vi "Brute Force Dark Current Primary Logic Body.vi"(0 "Barcodes in":string[](array[string]), 1 "stop":bool, 2 "Data Pin in":refnum<k21>, 3 "Sync Pin in":refnum<k21>, 4 "Write Pin in":refnum<k21>, 5 "Clear Pin in":refnum<k21>, 6 "Number of Tubes":i32, 7 "Channel #":i32, 8 "Trip Count":dbl) -> (10 "Actual Voltage Level (V)":dbl format="%#_13g", 11 "Individual Tube Current (Nano Amps)":dbl[](array[numeric]), 12 "Actual Current Limit (nA)":dbl format="%#_13g", 13 "Mesurnment Iteration":i32, 14 "Power Supply Trip":bool, 15 "Data Pin out":refnum<k21>, 16 "Sync Pin out":refnum<k21>, 17 "Write Pin out":refnum<k21>, 18 "Clear Pin out":refnum<k21>, 19 "Failed Tubes":string[](array[string]))   [LabVIEW 2020]
uses:
  <instrlib>/CAEN PSM/CAEN PSM.lvlib
panel:
  out "BoardHandle out":T1
  out "error out":errorcluster
  in  "VISA Refnum in":refnum<visa-resource-name>
  # "Pin in"
  # "Pin out"
  # "No pin"
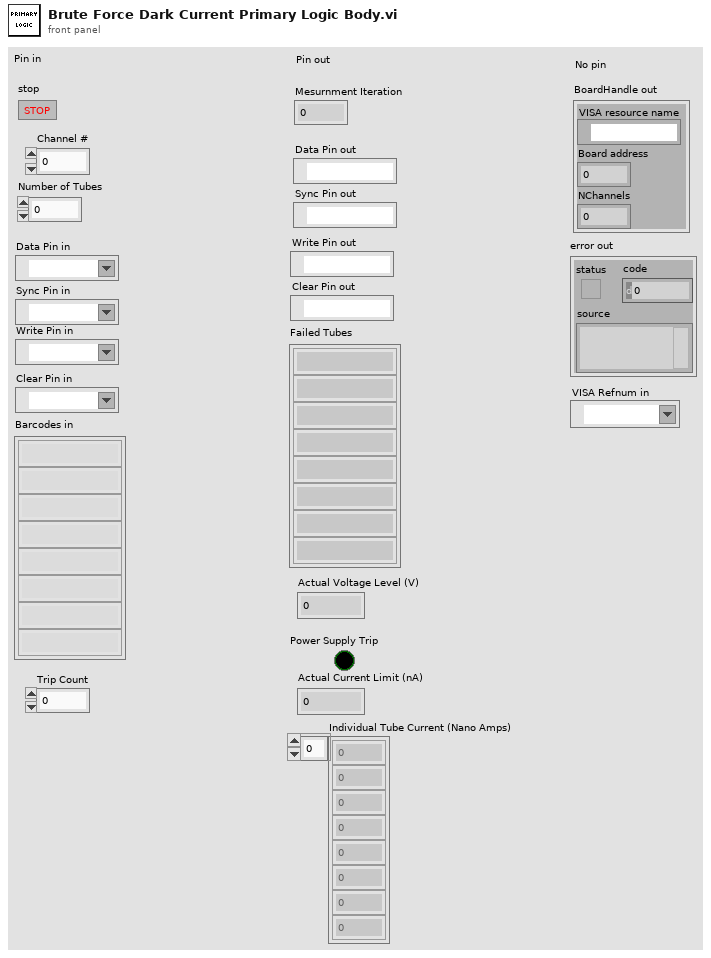
[diagram p1: front panel]
types:
  T1 = cluster{"VISA resource name":refnum<visa-resource-name>, "Board address":u8, "NChannels":u8}
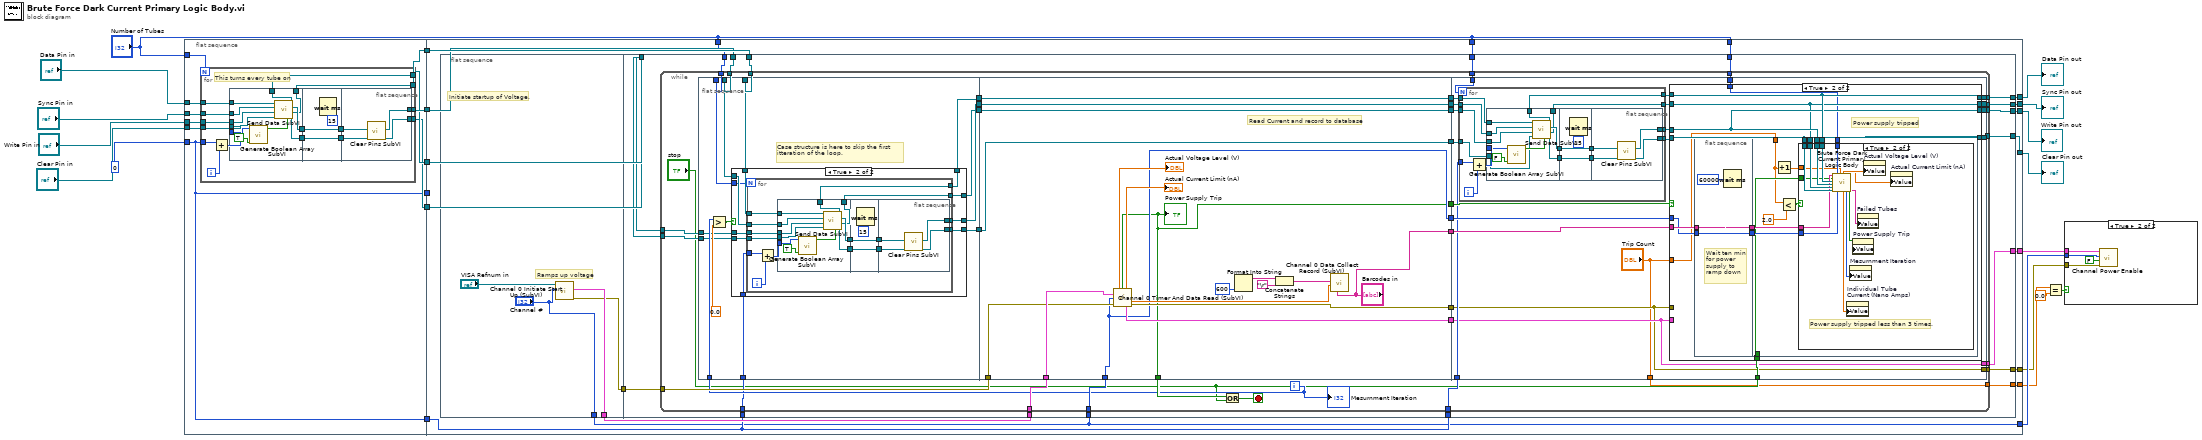
[diagram p0: block diagram]
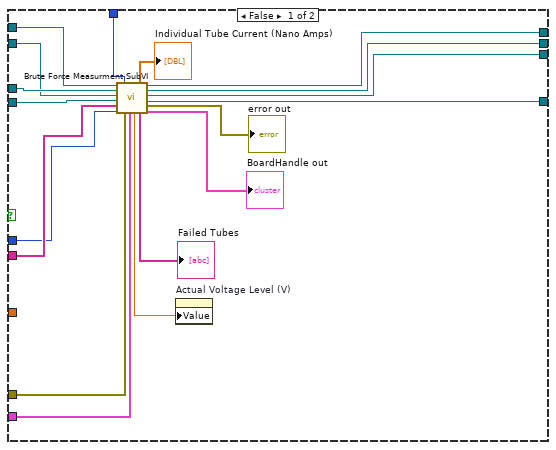
[diagram p4: hidden frame]
diagram:
  n1 = flat-sequence {
    tunnel: 0 ("First Tube #") -> [w23]
    tunnel: "Number of Tubes" -> [w29]
    tunnel: "Data Pin in" -> [w32]
    tunnel: "Sync Pin in" -> [w31]
    tunnel: "Write Pin in" -> [w30]
    tunnel: [w23] -> w22
    tunnel: "Clear Pin in" -> [w28]
    tunnel: [w27] -> w16
    tunnel: [w26] -> w15
    tunnel: [w25] -> w14
    tunnel: [w24] -> w13
    tunnel: [w23] -> w11
    tunnel: w22 -> [w70]
    tunnel: "Number of Tubes" -> [w83]
    tunnel: w16 -> [w80]
    tunnel: w15 -> [w79]
    tunnel: w14 -> [w78]
    tunnel: w13 -> [w77]
    tunnel: "Number of Tubes" -> [w82]
    tunnel: "Number of Tubes" -> [w76]
    tunnel: w11 -> [_]
    tunnel: [w74] -> w10
    tunnel: [w73] -> w9
    tunnel: [w72] -> w8
    tunnel: [w71] -> w7
    tunnel: [w69] -> w6
    tunnel: [w68] -> w5
    tunnel: [w67] -> w4
    tunnel: [w66] -> w2
    frame #0 {
      n2 = for {
        N: w29 -> [_]
        tunnel: w32 -> [w47]
        tunnel: w31 -> [w46]
        tunnel: w30 -> [w45]
        tunnel: [w44] -> w26
        tunnel: [w43] -> w24
        tunnel: [w42] -> w25
        tunnel: [w41] -> w27
        tunnel: w23 -> [w38]
        tunnel: w28 -> [w37]
        i -> [w39]
        # "This turns every tube on"
        n3 = Add(x=w38, y=w39) -> (x+y=w40:i32)
        n4 = flat-sequence {
          tunnel: w40 -> [w56]
          tunnel: w47 -> [w55]
          tunnel: w46 -> [w54]
          tunnel: w45 -> [w53]
          tunnel: [w52] -> w36
          tunnel: [w51] -> w34
          tunnel: [w50] -> w42
          tunnel: [w49] -> w41
          tunnel: w37 -> [w48]
          tunnel: w36 -> [w61]
          tunnel: [w61] -> w35
          tunnel: w34 -> [w60]
          tunnel: [w60] -> w33
          tunnel: w35 -> [w65]
          tunnel: w33 -> [w64]
          tunnel: [w63] -> w44
          tunnel: [w62] -> w43
          frame #0 {
            n5 = call "Generate Boolean Array SubVI.vi"("Activate: 1\nDeactivate: 0"=TRUE, "Tube"=w56) -> ("Boolean array"=w57:bool[])  [unwired: 9 in]
            n6 = call "Send Data SubVI.vi"("Data Pin Task In"=w55, "Sync Pin Task In"=w54, "Write Pin Task In"=w53, "Clear Pin Task In"=w48, "Data"=w57) -> ("Data Pin Task Out"=w49:refnum<k21>, "Sync Pin Task Out"=w52:refnum<k21>, "Write Pin Task Out"=w50:refnum<k21>, "Clear Pin Task Out"=w51:refnum<k21>)  [unwired: 1 in]
          }
          frame #1 {
            n7 = Wait (ms)(milliseconds to wait=u32 15) -> ()  [unwired: 1 out]
          }
          frame #2 {
            n8 = call "Clear Pins SubVI.vi"("Clear Pin Task In"=w64, "Sync Pin Task In"=w65) -> ("Clear Pin Task Out"=w62:refnum<k21>, "Sync Pin Task Out"=w63:refnum<k21>)  [unwired: 8 in]
          }
        }
      }
    }
    frame #1 {
      n9 = flat-sequence {
        tunnel: ["Channel #"] -> w69
        tunnel: [w86] -> w81
        tunnel: [w84] -> w75
        tunnel: w83 -> [w106]
        tunnel: w70 -> [w105]
        tunnel: w82 -> [w104]
        tunnel: w69 -> [w103]
        tunnel: w81 -> [w102]
        tunnel: w80 -> [w101]
        tunnel: w79 -> [w100]
        tunnel: w78 -> [w99]
        tunnel: w77 -> [w98]
        tunnel: w76 -> [w97]
        tunnel: w75 -> [w96]
        tunnel: [w95] -> w71
        tunnel: [w94] -> w72
        tunnel: [w93] -> w73
        tunnel: [w92] -> w74
        tunnel: w70 -> [w91]
        tunnel: [w90] -> w68
        tunnel: [w89] -> w67
        tunnel: [w88] -> w66
        frame #0 {
          # "Ramps up voltage"
          # "Initiate startup of Voltage."
          n10 = call "Channel 0 Initiate Start Up (SubVI).vi"("Channel # in"="Channel #", "VISA Refnum in"="VISA Refnum in") -> ("error out"=w84:errorcluster, "BoardHandle out"=w86:T1)  [unwired: 8 in]
        }
        frame #1 {
          n11 = while {
            tunnel: w106 -> [w142]
            tunnel: w105 -> [w141]
            tunnel: w104 -> [w140]
            tunnel: w103 -> [w139]
            tunnel: w102 -> [w138]
            tunnel: w101 -> [w137]
            tunnel: w100 -> [w136]
            tunnel: w99 -> [w135]
            tunnel: w98 -> [w134]
            tunnel: w97 -> [w125]
            tunnel: w96 -> [w120]
            tunnel: [w119] -> w95
            tunnel: [w118] -> w94
            tunnel: [w117] -> w93
            tunnel: [w116] -> w92
            tunnel: w91 -> [w112]
            tunnel: [w109] -> w90
            tunnel: [w108] -> w89
            tunnel: [w107] -> w88
            i -> [w113]
            stop <- w114 stop-if-true
            n12 = flat-sequence {
              tunnel: w113 -> [w153]
              tunnel: w137 -> [w152]
              tunnel: w136 -> [w151]
              tunnel: w135 -> [w150]
              tunnel: w134 -> [w149]
              tunnel: [w148] -> w132
              tunnel: [w147] -> w130
              tunnel: [w146] -> w128
              tunnel: [w145] -> w126
              tunnel: w125 -> [w144]
              tunnel: w112 -> [w143]
              tunnel: w139 -> [w204]
              tunnel: w138 -> [w207]
              tunnel: [w215] -> w133
              tunnel: w132 -> [w215]
              tunnel: [w214] -> w131
              tunnel: w130 -> [w214]
              tunnel: [w213] -> w129
              tunnel: w128 -> [w213]
              tunnel: [w212] -> w127
              tunnel: w126 -> [w212]
              tunnel: [w211] -> w124
              tunnel: [w204] -> w123
              tunnel: [w209] -> w122
              tunnel: ["Barcodes in"] -> w121
              tunnel: w120 -> [w206]
              tunnel: [w203] -> w115
              tunnel: [w203] -> w111
              tunnel: w142 -> [w240]
              tunnel: [w239] -> w119
              tunnel: [w238] -> w118
              tunnel: [w237] -> w117
              tunnel: [w236] -> w116
              tunnel: w121 -> [w242]
              tunnel: w122 -> [w223]
              tunnel: w123 -> [w241]
              tunnel: w124 -> [w222]
              tunnel: w127 -> [w229]
              tunnel: w129 -> [w230]
              tunnel: w131 -> [w231]
              tunnel: w133 -> [w232]
              tunnel: w140 -> [w234]
              tunnel: w141 -> [w233]
              tunnel: w111 -> [w235]
              tunnel: "stop" -> [w224]
              tunnel: [w223] -> w109
              tunnel: [w222] -> w108
              tunnel: ["Trip Count"] -> w107
              frame #0 {
                # "Case structure is here to skip the first itteration of the loop."
                n13 = Greater?(x=w153, y=0.0) -> (0:w155:bool)
                n14 = case shown="True" w155 {
                  tunnel: w152 -> [w159 w169]
                  tunnel: w151 -> [w158 w168]
                  tunnel: w150 -> [w157 w167]
                  tunnel: w149 -> [w156 w166]
                  tunnel: [w159 w165] -> w148
                  tunnel: [w158 w164] -> w147
                  tunnel: [w157 w163] -> w146
                  tunnel: [w156 w162] -> w145
                  tunnel: w144 -> [_ w161]
                  tunnel: w143 -> [_ w160]
                  frame False {
                  }
                  frame True {
                    n15 = for {
                      N: w161 -> [_]
                      tunnel: w169 -> [w184]
                      tunnel: w168 -> [w183]
                      tunnel: w167 -> [w182]
                      tunnel: [w181] -> w164
                      tunnel: [w180] -> w162
                      tunnel: [w179] -> w163
                      tunnel: [w178] -> w165
                      tunnel: w160 -> [w175]
                      tunnel: w166 -> [w174]
                      i -> [w176]
                      n16 = Add(x=w175, y=w176) -> (x+y=w177:i32)
                      n17 = flat-sequence {
                        tunnel: w177 -> [w193]
                        tunnel: w184 -> [w192]
                        tunnel: w183 -> [w191]
                        tunnel: w182 -> [w190]
                        tunnel: [w189] -> w173
                        tunnel: [w188] -> w171
                        tunnel: [w187] -> w179
                        tunnel: [w186] -> w178
                        tunnel: w174 -> [w185]
                        tunnel: w173 -> [w198]
                        tunnel: [w198] -> w172
                        tunnel: w171 -> [w197]
                        tunnel: [w197] -> w170
                        tunnel: w172 -> [w202]
                        tunnel: w170 -> [w201]
                        tunnel: [w200] -> w181
                        tunnel: [w199] -> w180
                        frame #0 {
                          n18 = call "Generate Boolean Array SubVI.vi"("Activate: 1\nDeactivate: 0"=TRUE, "Tube"=w193) -> ("Boolean array"=w194:bool[])  [unwired: 9 in]
                          n19 = call "Send Data SubVI.vi"("Data Pin Task In"=w192, "Sync Pin Task In"=w191, "Write Pin Task In"=w190, "Clear Pin Task In"=w185, "Data"=w194) -> ("Data Pin Task Out"=w186:refnum<k21>, "Sync Pin Task Out"=w189:refnum<k21>, "Write Pin Task Out"=w187:refnum<k21>, "Clear Pin Task Out"=w188:refnum<k21>)  [unwired: 1 in]
                        }
                        frame #1 {
                          n20 = Wait (ms)(milliseconds to wait=u32 15) -> ()  [unwired: 1 out]
                        }
                        frame #2 {
                          n21 = call "Clear Pins SubVI.vi"("Clear Pin Task In"=w201, "Sync Pin Task In"=w202) -> ("Clear Pin Task Out"=w199:refnum<k21>, "Sync Pin Task Out"=w200:refnum<k21>)  [unwired: 8 in]
                        }
                      }
                    }
                  }
                }
              }
              frame #1 {
                # "Read Current and record to database"
                n22 = call "Channel 0 Timer And Data Read (SubVI).vi"("BoardHandle in"=w207, "Channel # in"=w204, "error in (no error)"=w206) -> ("Actual Voltage Level (V)"=→"Actual Voltage Level (V)":dbl, "Power Supply Trip"=w203:bool, "Actual Current Limit (nA)"=→"Actual Current Limit (nA)":dbl, "Array"=w210:dbl[], "BoardHandle out 2"=w209:T1, "error out"=w211:errorcluster)  [unwired: 7 in]
                "Power Supply Trip" <- w203
                n23 = Format Into String(600 ("input 1")) -> (resulting string=w219:string)  [unwired: 3 in, 1 out]
                n24 = Concatenate Strings(w219, "\r") -> (w220:string)
                n25 = call "Channel 0 Data Collect Record (SubVI).vi"("Barcodes"="Barcodes in", "Array"=w210, "String"=w220) -> ()  [unwired: 9 in]
              }
              frame #2 {
                n26 = for {
                  N: w234 -> [_]
                  tunnel: w232 -> [w257]
                  tunnel: w231 -> [w256]
                  tunnel: w230 -> [w255]
                  tunnel: [w254] -> w226
                  tunnel: [w253] -> w228
                  tunnel: [w252] -> w225
                  tunnel: w233 -> [w248]
                  tunnel: w229 -> [w247]
                  tunnel: [w251] -> w227
                  i -> [w249]
                  n27 = Add(x=w248, y=w249) -> (x+y=w250:i32)
                  n28 = flat-sequence {
                    tunnel: w250 -> [w266]
                    tunnel: w257 -> [w265]
                    tunnel: w256 -> [w264]
                    tunnel: w255 -> [w263]
                    tunnel: [w262] -> w246
                    tunnel: [w261] -> w244
                    tunnel: [w260] -> w252
                    tunnel: [w259] -> w251
                    tunnel: w247 -> [w258]
                    tunnel: w246 -> [w271]
                    tunnel: [w271] -> w245
                    tunnel: w244 -> [w270]
                    tunnel: [w270] -> w243
                    tunnel: w245 -> [w275]
                    tunnel: w243 -> [w274]
                    tunnel: [w273] -> w254
                    tunnel: [w272] -> w253
                    frame #0 {
                      n29 = call "Generate Boolean Array SubVI.vi"("Activate: 1\nDeactivate: 0"=FALSE, "Tube"=w266) -> ("Boolean array"=w267:bool[])  [unwired: 9 in]
                      n30 = call "Send Data SubVI.vi"("Data Pin Task In"=w265, "Sync Pin Task In"=w264, "Write Pin Task In"=w263, "Clear Pin Task In"=w258, "Data"=w267) -> ("Data Pin Task Out"=w259:refnum<k21>, "Sync Pin Task Out"=w262:refnum<k21>, "Write Pin Task Out"=w260:refnum<k21>, "Clear Pin Task Out"=w261:refnum<k21>)  [unwired: 1 in]
                    }
                    frame #1 {
                      n31 = Wait (ms)(milliseconds to wait=u32 15) -> ()  [unwired: 1 out]
                    }
                    frame #2 {
                      n32 = call "Clear Pins SubVI.vi"("Clear Pin Task In"=w274, "Sync Pin Task In"=w275) -> ("Clear Pin Task Out"=w272:refnum<k21>, "Sync Pin Task Out"=w273:refnum<k21>)  [unwired: 8 in]
                    }
                  }
                }
                n33 = case shown="True" w235 {
                  tunnel: w242 -> [w293 w299]
                  tunnel: w241 -> [w292 w298]
                  tunnel: w222 -> [w291 _]
                  tunnel: w240 -> [w290 w300]
                  tunnel: w223 -> [w287 _]
                  tunnel: [w286 w303] -> w239
                  tunnel: [w285 w302] -> w238
                  tunnel: [w284 w301] -> w237
                  tunnel: [w283 w304] -> w236
                  tunnel: w227 -> [w279 w304]
                  tunnel: w225 -> [w277 w301]
                  tunnel: w226 -> [w278 w302]
                  tunnel: w228 -> [w276 w303]
                  tunnel: w224 -> [_ w297]
                  tunnel: "Trip Count" -> [_ w294]
                  frame False {
                    n34 = call "Brute Force Measurment SubVI.vi"("Data Pin Task In"=w279, "Sync Pin Task In"=w278, "Write Pin Task In"=w277, "Clear Pin Task In"=w276, "Barcodes in"=w293, "Channel # in"=w292, "Number of Active tubes"=w290, "error in (no error)"=w291, "BoardHandle in"=w287) -> ("Actual Voltage Level (V) 2"=w289:dbl, "Individual Tube Current (Nano Amps)"=→"Individual Tube Current (Nano Amps)":dbl[], "Failed Tubes"=→"Failed Tubes":string[], "Data Pin Task Out"=w283:refnum<k21>, "Sync Pin Task Out"=w284:refnum<k21>, "Write Pin Task Out"=w285:refnum<k21>, "Clear Pin Task Out"=w286:refnum<k21>, "error out"=→"error out":errorcluster, "BoardHandle out"=→"BoardHandle out":T1)  [unwired: 2 in]
                    n35 = property on="Actual Voltage Level (V)" class="DigNum (strict)"("Value"=w289) -> ()  [unwired: 2 in, 2 out]
                  }
                  frame True {
                    # "Power supply tripped"
                    n36 = flat-sequence {
                      tunnel: w298 -> [w306]
                      tunnel: w299 -> [w307]
                      tunnel: [w307] -> w296
                      tunnel: [w306] -> w295
                      tunnel: w304 -> [w317]
                      tunnel: w303 -> [w316]
                      tunnel: w302 -> [w315]
                      tunnel: w301 -> [w314]
                      tunnel: w300 -> [w313]
                      tunnel: w297 -> [w310]
                      tunnel: w296 -> [w312]
                      tunnel: w295 -> [w311]
                      tunnel: w294 -> [w308]
                      frame #0 {
                        # "Wait ten min\nfor power \nsupply to \nramp down"
                        n37 = Wait (ms)(milliseconds to wait=u32 60000) -> ()  [unwired: 1 out]
                      }
                      frame #1 {
                        n38 = Increment(x=w308) -> (x+1=w309:dbl)
                        n39 = Less?(x=w308, y=2.0) -> (x < y?=w319:bool)
                        n40 = case shown="True" w319 {
                          tunnel: w317 -> [_ w334]
                          tunnel: w316 -> [_ w333]
                          tunnel: w315 -> [_ w332]
                          tunnel: w314 -> [_ w331]
                          tunnel: w313 -> [_ w330]
                          tunnel: w312 -> [_ w329]
                          tunnel: w311 -> [_ w328]
                          tunnel: w310 -> [_ w327]
                          tunnel: w309 -> [_ w326]
                          frame False {
                          }
                          frame True {
                            # "Power supply tripped less than 3 times."
                            n41 = call "Brute Force Dark Current Primary Logic Body.vi"("Barcodes in"=w329, "stop"=w327, "Data Pin in"=w334, "Sync Pin in"=w332, "Write Pin in"=w331, "Clear Pin in"=w333, "Number of Tubes"=w330, "Channel #"=w328, "Trip Count"=w326) -> ("Actual Voltage Level (V)"=w322:dbl, "Individual Tube Current (Nano Amps)"=w325:dbl[], "Actual Current Limit (nA)"=w321:dbl, "Mesurnment Iteration"=w324:i32, "Power Supply Trip"=w323:bool, "Failed Tubes"=w320:string[])  [unwired: 1 in, 4 out]
                            n42 = property on="Individual Tube \nCurrent (Nano Amps)" class="Arr (strict)"("Value"=w325) -> ()  [unwired: 2 in, 2 out]
                            n43 = property on="Mesurnment Iteration" class="DigNum (strict)"("Value"=w324) -> ()  [unwired: 2 in, 2 out]
                            n44 = property on="Power Supply Trip" class="Bool (strict)"("Value"=w323) -> ()  [unwired: 2 in, 2 out]
                            n45 = property on="Failed Tubes" class="Arr (strict)"("Value"=w320) -> ()  [unwired: 2 in, 2 out]
                            n46 = property on="Actual Voltage Level (V)" class="DigNum (strict)"("Value"=w322) -> ()  [unwired: 2 in, 2 out]
                            n47 = property on="Actual Current Limit (nA)" class="DigNum (strict)"("Value"=w321) -> ()  [unwired: 2 in, 2 out]
                          }
                        }
                      }
                    }
                  }
                }
              }
            }
            n48 = Or(x=w115, y="stop") -> (x .or. y?=w114:bool)
            "Mesurnment Iteration" <- w113
          }
        }
      }
    }
  }
  n49 = Equal?(x=w2, y=0.0) -> (x = y?=w3:bool)
  n50 = case shown="True" w3 {
    tunnel: w6 -> [_ w337]
    tunnel: w5 -> [_ w336]
    tunnel: w4 -> [_ w335]
    frame False {
    }
    frame True {
      n51 = call <instrlib>:"Channel Power Enable.vi"("error in (no error)"=w335, "Enable (OFF)"=FALSE, "Channel (0)"=w337, "BoardHandle"=w336) -> ()  [unwired: 6 in, 2 out]
    }
  }
  "Data Pin out" <- w10
  "Sync Pin out" <- w9
  "Write Pin out" <- w8
  "Clear Pin out" <- w7
